vi "Rd_all.vi"(8 "error in (no error)":errorcluster, 9 "Name in":string, 10 "machine name (\"\":  open local reference)":string, 11 "Vi path":path) -> (0 "error out":errorcluster, 2 "Rd_all Array":variant[](array[variant]), 3 "Number of  Tuples":i32)   [LabVIEW 2015]
doc: "Reads all tuple with \"Name in\" name, If a VI path is provided and eventually a machine name each tuple is processed using that VI on that machine."
uses:
  LI_states.ctl
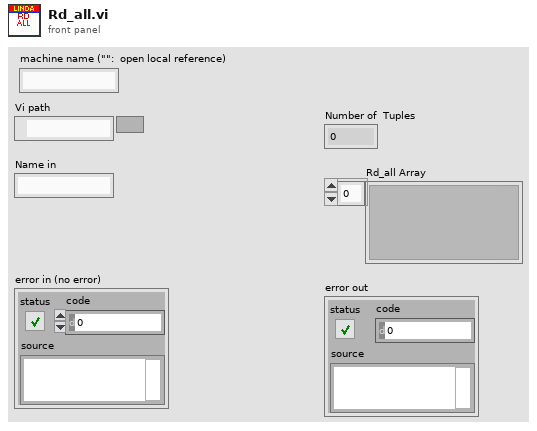
[diagram p1: front panel]
types:
  T1 = typedef "LI_states.ctl" = enum16{"Out", "In", "Rd", "Inp", "Rdp", "Init", "Cleanup", "RdAll"}
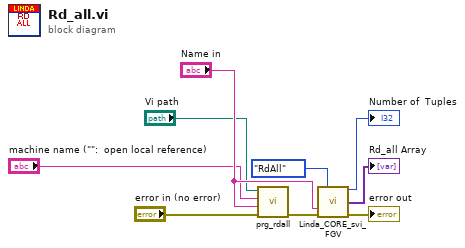
[diagram p0: block diagram]
diagram:
  n1 = call "prg_rdall.vi"("error in (no error)"="error in (no error)", "Name"="Name in", "machine name (\"\":  open local reference)"="machine name (\"\":  open local reference)", "vi path"="Vi path") -> ("error out"=w4:errorcluster)  [unwired: 7 in]
  n2 = call "Linda_CORE_svi_FGV.vi"("OP"=LI_states."RdAll", "Name in"="Name in", "error in (no error)"=w4) -> ("Number of  Tuples"=→"Number of  Tuples":i32, "Rd_all Array"=→"Rd_all Array":variant[], "error out"=→"error out":errorcluster)  [unwired: 8 in, 2 out]
